vi "TDMS.SetMetadata.Generic.vi"(8 "error in (no error)":errorcluster, 10 "MetaData":T1(array[cluster]), 11 "Data":path) -> (0 "error out":errorcluster)   [LabVIEW 2014, in "ParametericRoutines.lvlib"]
doc: "- Set Property Name w/ function NameOf() which returns the name of the metadata variable you are logging.\n- Set Property Value w/ function Str() to convert the value of the metadata variable to a sting."
uses:
  ParametericRoutines.lvlib
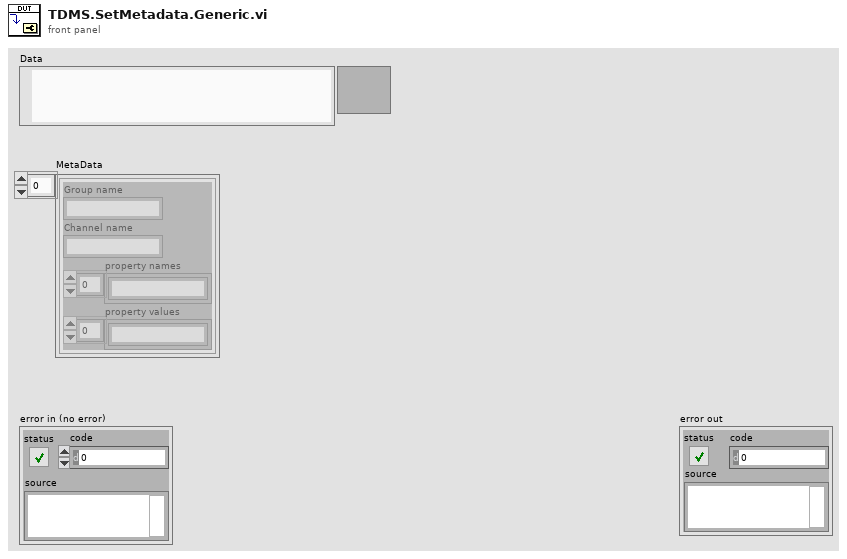
[diagram p1: front panel]
types:
  T1 = cluster{"Group name":string, "Channel name":string, "property names":string[], "property values":string[]}[]
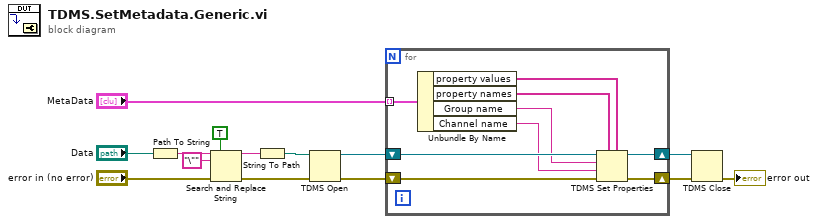
[diagram p0: block diagram]
diagram:
  n1 = Path To String(path="Data") -> (string=w13:string)
  n2 = Search and Replace String(replace all?=TRUE ("replace all? (F)"), input string=w13, search string="\"", error in="error in (no error)") -> (result string=w14:string, error out=w8:errorcluster)  [unwired: 4 in, 2 out]
  n3 = String To Path(string=w14) -> (path=w9:path)
  n4 = TDMS Open(8:w8, 11:w9) -> (0:w4:errorcluster, 3:w5:refnum<k34>)  [unwired: 5 in]
  n5 = for {
    shift-right: [w21] -> w3
    shift-left: w5 -> [w23]
    shift-right: [w20] -> w2
    shift-left: w4 -> [w22]
    tunnel: "MetaData" -> [w19] mode=indexing
    n6 = Unbundle By Name(w19) -> ("property values"=w17:string[], "property names"=w18:string[], "Group name"=w16:string, "Channel name"=w15:string)
    n7 = TDMS Set Properties(5:w17, 7:w18, 8:w22, 9:w15, 10:w16, 11:w23) -> (0:w20:errorcluster, 3:w21:refnum<k34>)  [unwired: 2 out]
  }
  n8 = TDMS Close(8:w2, 11:w3) -> (0:→"error out":errorcluster)  [unwired: 1 out]
